vi "Check Firmware Compatibility.vi"(8 "error in (no error)":errorcluster, 11 "PLBB in":refnum<class "PL BlackBox Modbus Client.lvclass">) -> (0 "error out":errorcluster, 3 "PLBB out":refnum<class "PL BlackBox Modbus Client.lvclass">)   [LabVIEW 2015, in "PL BlackBox Modbus Client.lvclass"]
doc: "Checks if the software is compatible with the firmware."
uses:
  PL BlackBox Modbus Client.lvclass
  PL BlackBox Modbus Client.lvclass/PL BlackBox Modbus Client.ctl
  <vilib>/plasmapper/PL Modbus Client/PL Modbus Client.lvclass
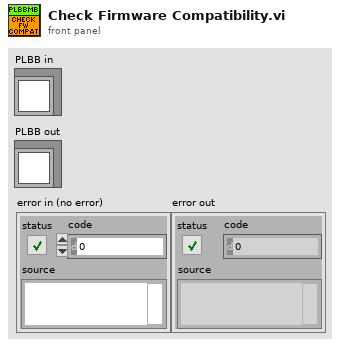
[diagram p1: front panel]
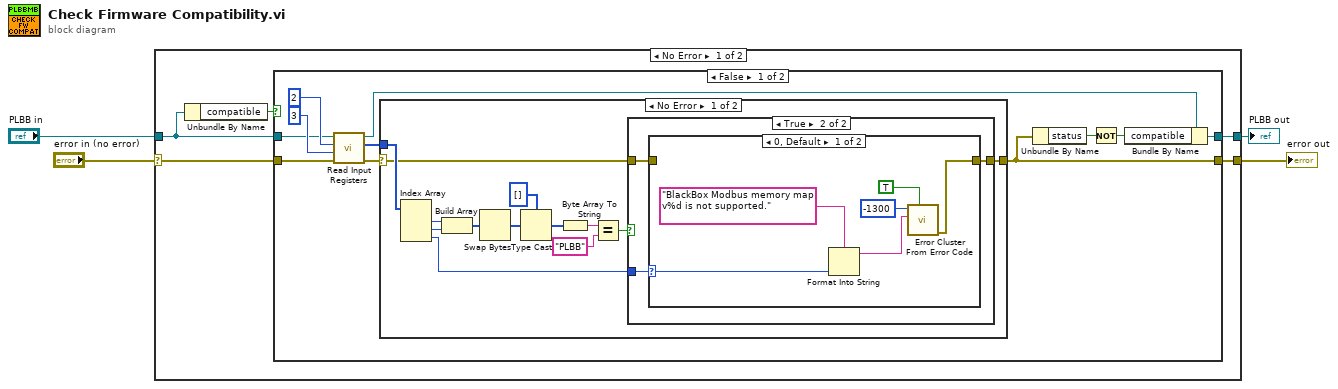
[diagram p0: block diagram]
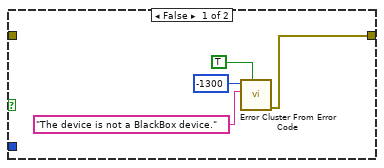
[diagram p2: hidden frame]
diagram:
  n1 = case shown="No Error" "error in (no error)" {
    selector: "error in (no error)" -> [w5 w51]
    tunnel: [w9 w51] -> w4
    tunnel: [w8 w52] -> w3
    tunnel: "PLBB in" -> [w7 w52]
    frame No Error {
      n2 = Unbundle By Name(w7) -> ("compatible"=w6:bool)
      n3 = case shown="False" w6 {
        tunnel: [w12 w49] -> w9
        tunnel: w5 -> [w20 w49]
        tunnel: [w14 w50] -> w8
        tunnel: w7 -> [w17 w50]
        frame False {
          n4 = call <vilib>:"Read Input Registers.vi"("error in (no error)"=w20, "number of input registers"=u16 3 ("address"), "address"=u16 2, "MODBUS in"=w17) -> ("error out"=w15:errorcluster, "values"=w16:u16[], "MODBUS out"=w13:refnum<class "PL BlackBox Modbus Client.lvclass">)  [unwired: 5 in]
          n5 = case shown="No Error" w15 {
            selector: w15 -> [w23 w48]
            tunnel: w16 -> [w33 _]
            tunnel: [w21 w48] -> w12
            frame No Error {
              n6 = Index Array(array=w33) -> (element #1=w32:u16, element #2=w31:u16, element #3=w22:u16)  [unwired: 3 in]
              n7 = Build Array(w32, w31) -> (w30:u16[])
              n8 = Swap Bytes(anything=w30) -> (byte swapped=w28:u16[])
              n9 = Type Cast(type=u8[] [], x=w28) -> (*(type *) &x=w27:u8[])
              n10 = Byte Array To String(unsigned byte array=w27) -> (string=w26:string)
              n11 = Equal?(x=w26, y="PLBB") -> (x = y?=w24:bool)
              n12 = case shown="True" w24 {
                tunnel: w23 -> [_ w38]
                tunnel: w22 -> [_ w39]
                tunnel: [w34 w40] -> w21
                frame False {
                  n13 = call <vilib>:"Error Cluster From Error Code.vi"("show call chain? (False)"=TRUE, "error message (\"\")"="The device is not a BlackBox device." ("error message (\"\")"), "error code (0)"=-1300) -> ("error out"=w34:errorcluster)  [unwired: 6 in]
                }
                frame True {
                  n14 = case shown="0, Default" w39 {
                    selector: w39 -> [w42 _]
                    tunnel: [w44 w47] -> w40
                    tunnel: w38 -> [_ w47]
                    frame 0, Default {
                      n15 = Format Into String(format string="BlackBox Modbus memory map v%d is not supported." ("error message (\"\")"), w42) -> (resulting string=w41:string)  [unwired: 2 in, 1 out]
                      n16 = call <vilib>:"Error Cluster From Error Code.vi"("show call chain? (False)"=TRUE, "error message (\"\")"=w41, "error code (0)"=-1300) -> ("error out"=w44:errorcluster)  [unwired: 6 in]
                    }
                    frame 1 {
                    }
                  }
                }
              }
            }
            frame Error {
            }
          }
          n17 = Unbundle By Name(w12) -> ("status"=w11:bool)
          n18 = Not(x=w11) -> (.not. x?=w10:bool)
          n19 = Bundle By Name(cluster=w13, "compatible"=w10) -> (w14:refnum<class "PL BlackBox Modbus Client.lvclass">)
        }
        frame True {
        }
      }
    }
    frame Error {
    }
  }
  "error out" <- w4
  "PLBB out" <- w3
